vi "ConnectedStatus.vi"(8 "error in (no error)":errorcluster, 11 "PacificPowerSource in":refnum<class "PacificPowerSource.lvclass">) -> (0 "error out":errorcluster, 2 "Any Connections":bool, 3 "PacificPowerSource out":refnum<class "PacificPowerSource.lvclass">)   [LabVIEW 2018, in "AcPwrPlugins.lvlib" / "PacificPowerSource.lvclass"]
uses:
  PacificPowerSource.lvclass
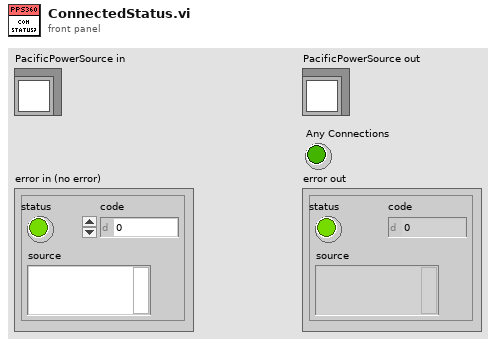
[diagram p1: front panel]
types:
  T1 = typedef "AcPwrPlugins.lvlib/PacificPowerSource.lvclass/DeviceSettings.ctl" = cluster{"Handle":string, "Connected":bool, "Source Limits and Range":cluster{"Frequency Minimum (45 Hz)":dbl, "Frequency Maximum (1200 Hz)":dbl, "Voltage Maximum (V)":dbl, "Voltage Minimum (V)":dbl, "Current Limit (40A)":dbl, "Range Control (0: Auto)":u16, "Initial Voltage (0V)":u16, "Frequency Range (600Hz)":u16, "Frequency (45Hz)":dbl}, "Clear Device (F)":bool, "Configure Output":cluster{"Coupling  (0: Direct)":u16, "Form (3: Three)":u16}, "btnIdQuery":bool, "btnReset":bool, "Waveform":cluster{"Voltage Level (V)":dbl, "Phase (Degrees)":i32, "Channel Name (1: A)":u16, "Waveform (1: Sine)":u16, "Petcentage Of Voltages for \nArbitrary Wavefrom":dbl[]}[], "Impedance Parameters (off, 0.00)":cluster{"State":bool, "Impedance":dbl}, "Program Number (0)":i32, "Transient Execution (F)":bool, "OutputEnabled":bool, "Measurement Complete Time (ms)":u32}[]
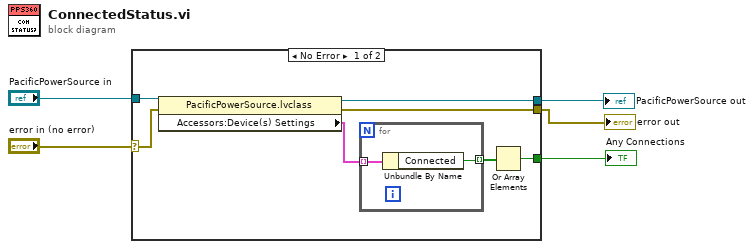
[diagram p0: block diagram]
diagram:
  n1 = case shown="No Error" "error in (no error)" {
    selector: "error in (no error)" -> [w11 w15]
    tunnel: "PacificPowerSource in" -> [w12 w16]
    tunnel: [w10 w16] -> w3
    tunnel: [w7 w15] -> w2
    tunnel: [w6 _] -> w1
    frame No Error {
      n2 = property class="PacificPowerSource.lvclass"(reference=w12, error in=w11) -> (reference out=w10:refnum<class "PacificPowerSource.lvclass">, error out=w7:errorcluster, "Accessors:Device(s) Settings"=w9:T1)
      n3 = for {
        tunnel: w9 -> [w14] mode=indexing
        tunnel: [w13] -> w8 mode=indexing
        n4 = Unbundle By Name(w14) -> ("Connected"=w13:bool)
      }
      n5 = Or Array Elements(Boolean array=w8) -> (logical OR=w6:bool)
    }
    frame Error {
    }
  }
  "error out" <- w2
  "PacificPowerSource out" <- w3
  "Any Connections" <- w1
